vi "Stop2.vi"(8 "Template":path, 9 "Imaginea":path) -> (3 "Snap - Right":T1(plugin-control), 10 "y":sgl, 11 "x":sgl)   [LabVIEW 2015]
panel:
  out "element":T2
  out "Image":T1(plugin-control)
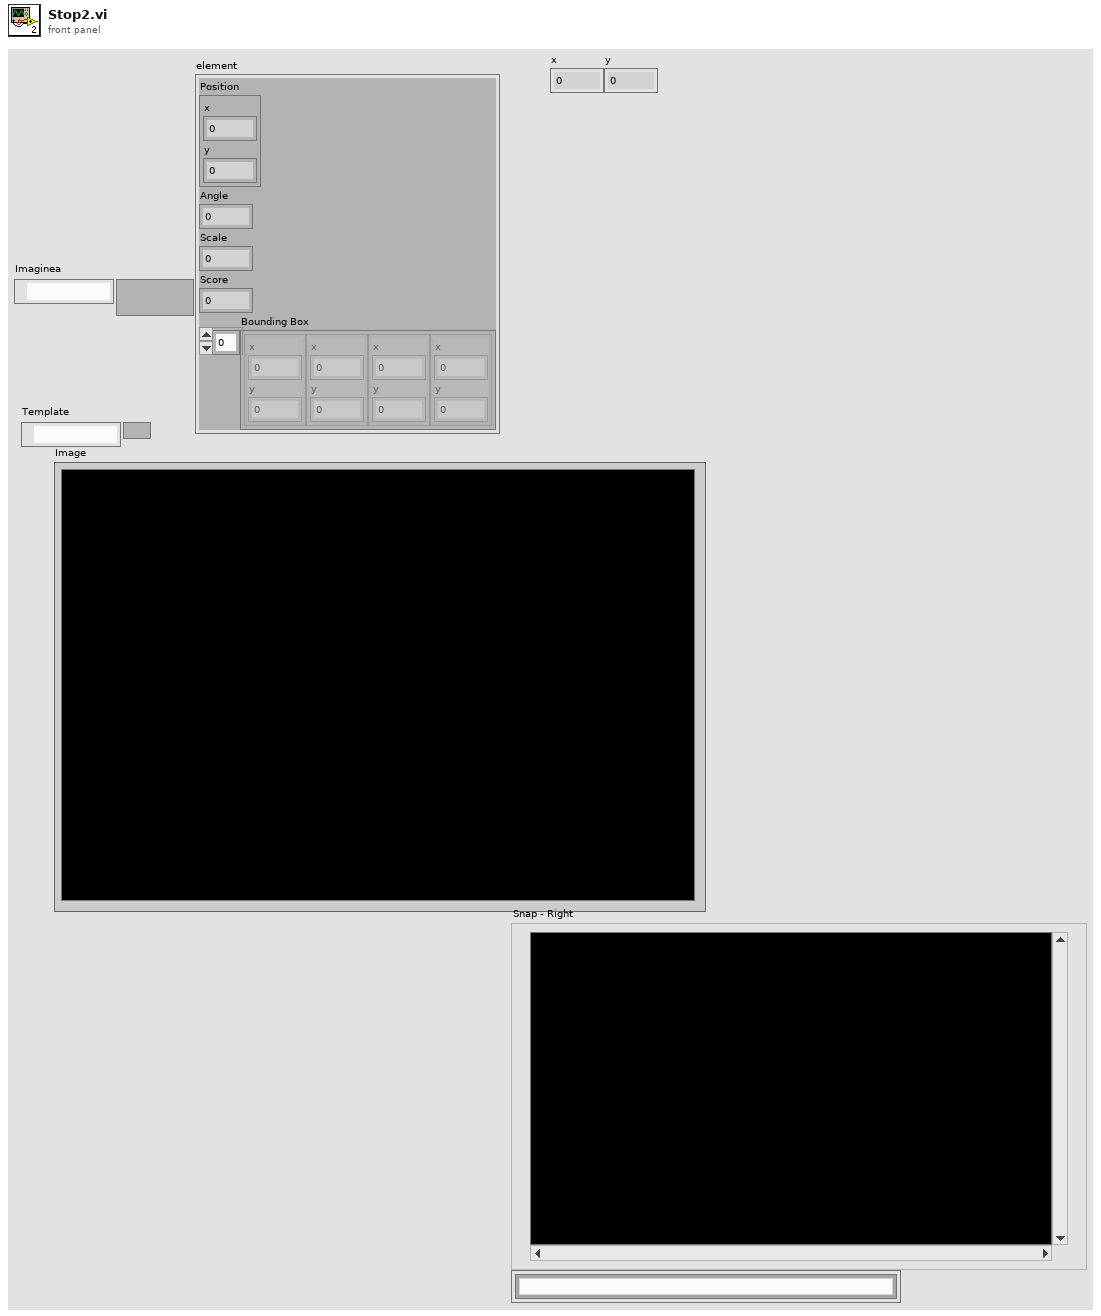
[diagram p1: front panel]
types:
  T1 = typedef "IMAQ Image.ctl" = refnum<image>
  T2 = cluster{"Position":cluster{"x":sgl, "y":sgl}, "Angle":sgl, "Scale":sgl, "Score":sgl, "Bounding Box":cluster{"x":sgl, "y":sgl}[]}
  T3 = cluster{"Position":cluster{"x":sgl, "y":sgl}, "Angle":sgl, "Scale":sgl, "Score":sgl, "Bounding Box":cluster{"x":sgl, "y":sgl}[]}[]
  T4 = typedef "LVPoint32TypeDef.ctl" = cluster{"Horizontal":i32, "Vertical":i32}
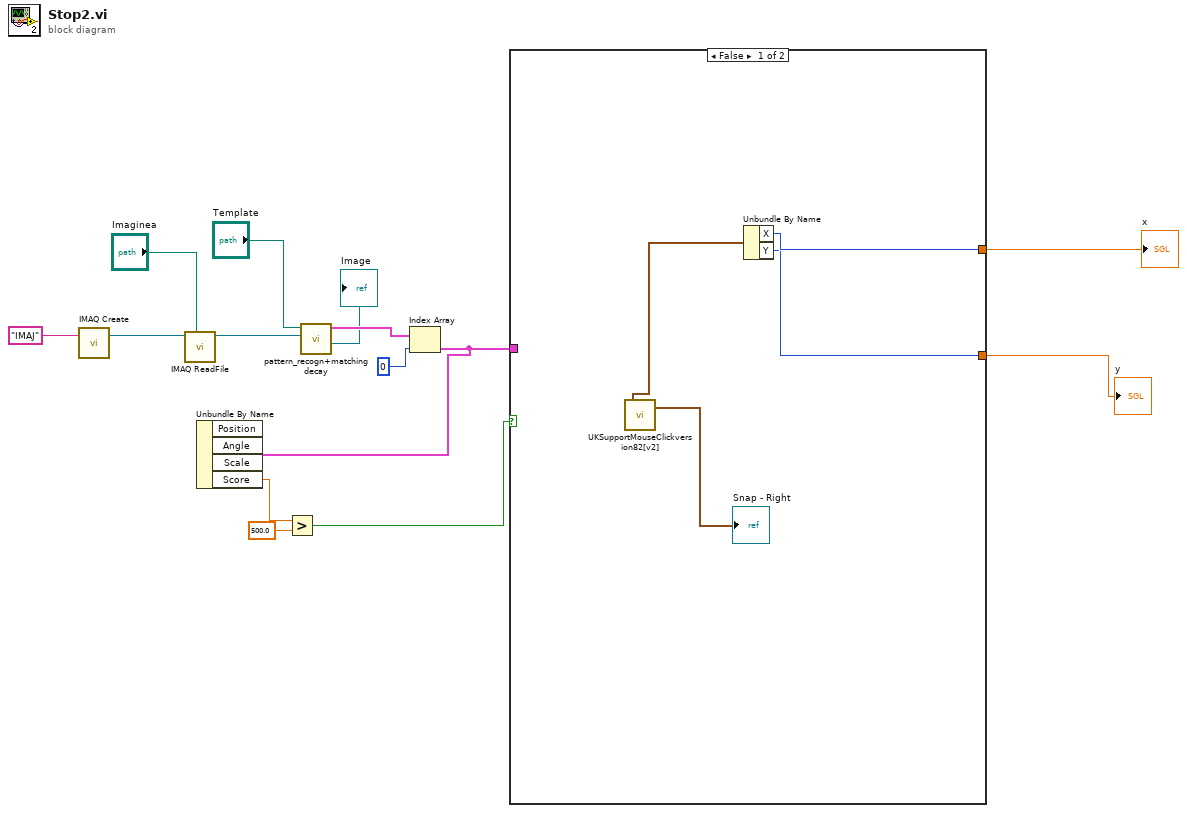
[diagram p0: block diagram]
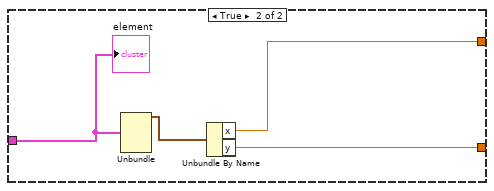
[diagram p2: hidden frame]
diagram:
  n1 = call "IMAQ Create"("Image Name"="IMAJ") -> ("New Image"=w14:T1)  [unwired: 4 in, 1 out]
  n2 = call "IMAQ ReadFile"("File Path"="Imaginea", "Image"=w14) -> ("Image Out"=w11:T1)  [unwired: 5 in, 4 out]
  n3 = call "pattern_recogn+matching decay.vi"("Image Out"=w11, "Path 3"="Template") -> ("Image"=→"Image":T1, "Matches (pixel)"=w9:T3)  [unwired: 7 in, 1 out]
  n4 = Index Array(array=w9, index=0) -> (element=w6:T2)
  n5 = Unbundle By Name(w6) -> ("Score"=w5:sgl)  [unwired: 3 out]
  n6 = Greater?(x=w5, y=sgl 500.0) -> (0:w3:bool)
  n7 = case shown="False" w3 {
    tunnel: w6 -> [_ w22]
    tunnel: [w18 w20] -> w2
    tunnel: [w17 w19] -> w1
    frame False {
      n8 = call "UKSupportMouseClickversion82[v2].vi"() -> ("Last Mouse Position:All Elements"=w16:cluster{"X":i32, "Y":i32}, "Coords"=→"Snap - Right":T4)  [unwired: 1 in]
      n9 = Unbundle By Name(w16) -> ("X"=w18:i32, "Y"=w17:i32)
    }
    frame True {
      n10 = Unbundle(w22) -> ("Position"=w21:cluster{"x":sgl, "y":sgl})  [unwired: 4 out]
      n11 = Unbundle By Name(w21) -> ("x"=w20:sgl, "y"=w19:sgl)
      "element" <- w22
    }
  }
  "x" <- w2
  "y" <- w1
